vi "display parameters.vi"(0 "LineCCD in":refnum<class "LineCCD.lvclass">, 5 "input cluster":T1, 11 "error in (no error)":errorcluster) -> (3 "y_min":dbl, 4 "LineCCD out":refnum<class "LineCCD.lvclass">, 6 "y_mean":dbl, 8 "A_g":dbl, 10 "STD":dbl, 14 "x_0":dbl, 15 "error out":errorcluster)   [LabVIEW 2012, in "LineCCD.lvclass"]
uses:
  LineCCD.lvclass
  fitting parameters.ctl
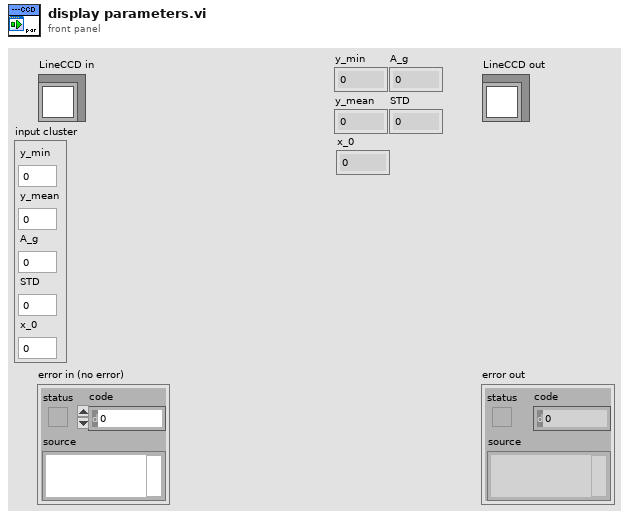
[diagram p1: front panel]
types:
  T1 = typedef "LineCCD.lvclass/fitting parameters.ctl" = cluster{"y_min":dbl, "y_mean":dbl, "A_g":dbl, "STD":dbl, "x_0":dbl}
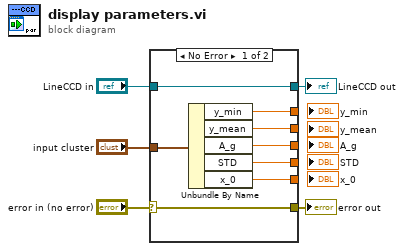
[diagram p0: block diagram]
diagram:
  n1 = case shown="No Error" "error in (no error)" {
    selector: "error in (no error)" -> [w13 w15]
    tunnel: [w13 w15] -> w4
    tunnel: [w12 w14] -> w2
    tunnel: "LineCCD in" -> [w12 w14]
    tunnel: [w11 _] -> _
    tunnel: [w10 _] -> _
    tunnel: [w9 _] -> _
    tunnel: [w8 _] -> _
    tunnel: [w7 _] -> _
    tunnel: "input cluster" -> [w6 _]
    frame No Error {
      n2 = Unbundle By Name(w6) -> ("y_min"=w11:dbl, "y_mean"=w10:dbl, "A_g"=w9:dbl, "STD"=w8:dbl, "x_0"=w7:dbl)
    }
    frame Error {
    }
  }
  "error out" <- w4
  "LineCCD out" <- w2
